vi "Collect Data1D.vi"(8 "error in (no error)":errorcluster, 10 "Data1D in":refnum<class "Data1D.lvclass">, 11 "AbstractCollector1D in":refnum<class "AbstractCollector1D.lvclass">) -> (0 "error out":errorcluster, 2 "finished?":bool=TRUE, 3 "AbstractCollector1D out":refnum<class "AbstractCollector1D.lvclass">)   [LabVIEW 2014, in "AbstractCollector1D.lvclass"]
uses:
  AbstractCollector1D.lvclass
  Model/Data/Data1D/Data1D.lvclass
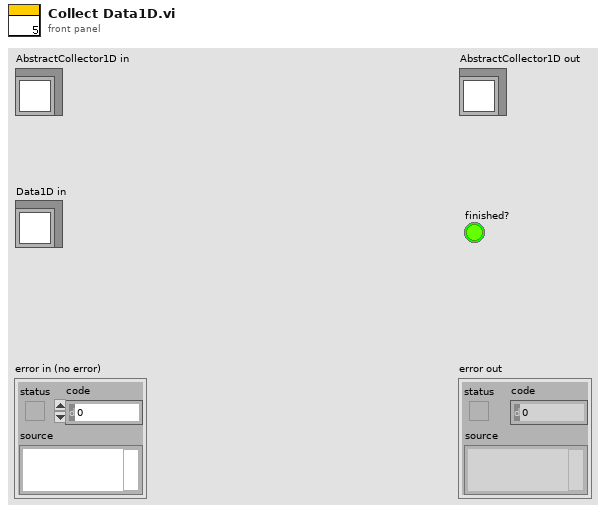
[diagram p1: front panel]
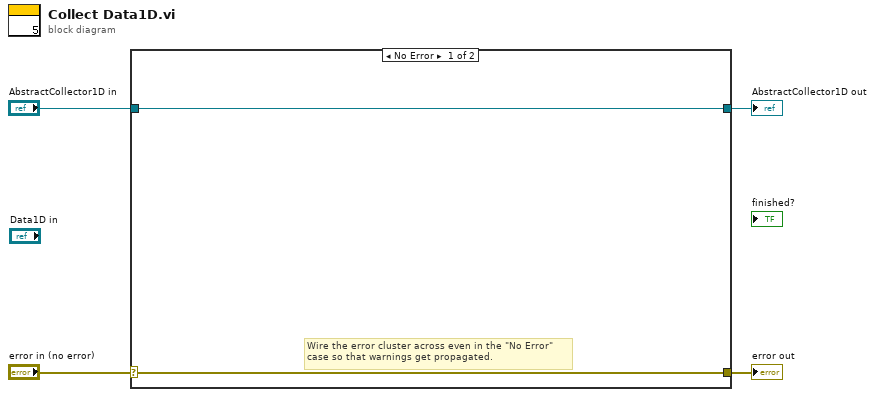
[diagram p0: block diagram]
diagram:
  n1 = case shown="No Error" "error in (no error)" {
    selector: "error in (no error)" -> [w5 w8]
    tunnel: [w5 w8] -> w3
    tunnel: [w6 w7] -> w1
    tunnel: "AbstractCollector1D in" -> [w6 w7]
    frame No Error {
      # "Wire the error cluster across even in the \"No Error\"\ncase so that warnings get propagated."
    }
    frame Error {
    }
  }
  "error out" <- w3
  "AbstractCollector1D out" <- w1
